vi "Read Type.vi"(8 "Error In":errorcluster, 11 "Partial In":refnum<class "Partial.lvclass">) -> (0 "Error Out":errorcluster, 2 "Type":T1=enum."Unknown", 3 "Partial Out":refnum<class "Partial.lvclass">)   [LabVIEW 2018, in "Toolkit.lvlib" / "Nodes.lvlib" / "Partial.lvclass"]
doc: "Gets the Node type of an object. This is primarily used internally or when building custom compilers. This is more robust than using strings in case structures with the Get LV Class Name function, which is not available in older versions of LabVIEW.\n\n<B>Partial In/Out</B> - Represents a node in an Abstract Syntax Tree (AST) for a parsed Mustache template.\n\n<B>Type</B> - Indicates the node's type as an enum."
uses:
  Partial.lvclass
  Type Definitions/Types.ctl
  Nodes.lvlib
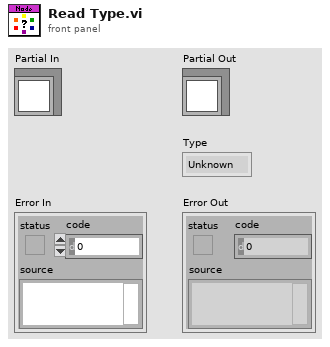
[diagram p1: front panel]
types:
  T1 = typedef "Toolkit.lvlib/Nodes.lvlib/Types.ctl" = enum16{"Comment", "Delimiter", "Partial", "Root", "Section", "Text", "Unknown", "Variable"}
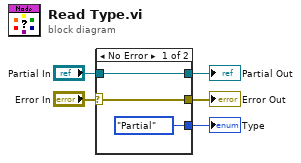
[diagram p0: block diagram]
diagram:
  n1 = case shown="No Error" "Error In" {
    selector: "Error In" -> [w8 w9]
    tunnel: [w8 w9] -> w4
    tunnel: "Partial In" -> [w7 w10]
    tunnel: [w7 w10] -> w2
    tunnel: [Types."Partial" ("Type") _] -> w1
    frame No Error {
    }
    frame Error {
    }
  }
  "Error Out" <- w4
  "Partial Out" <- w2
  "Type" <- w1
